vi "Inverse.vi"(10 "Inverse":dbl[][](array[numeric]), 11 "Inverse":bool caption="Scan") -> (2 "Array out":dbl[][](array[numeric]))   [LabVIEW 2018]
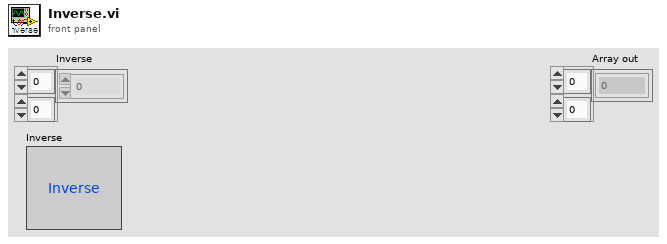
[diagram p1: front panel]
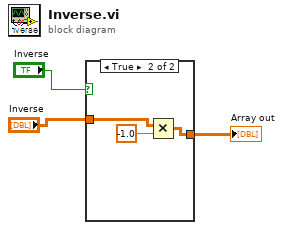
[diagram p0: block diagram]
diagram:
  n1 = case shown="True" "Inverse" {
    tunnel: "Inverse" -> [w4 w6]
    tunnel: [w4 w5] -> w1
    frame False {
    }
    frame True {
      n2 = Multiply(x=w6, y=-1.0) -> (x*y=w5:dbl[][])
    }
  }
  "Array out" <- w1
